vi "SetControlSpecific.vi"(7 "Dictionary":T2, 8 "error in (no error)":errorcluster, 9 "Font Info":T1, 10 "Target Language":string, 11 "Control Reference":refnum<vi>) -> (0 "error out":errorcluster, 3 "Control ref out":refnum<vi>)   [LabVIEW 2017, in "JKI Simple Localization.lvlib"]
uses:
  API/JKI Simple Localization.lvlib
  Definitions/Dictionary--Cluster.ctl
  Definitions/Private/FontCluster.ctl
  Definitions/Private/Phrase Dictionary.ctl
  Definitions/Private/Font Info.ctl
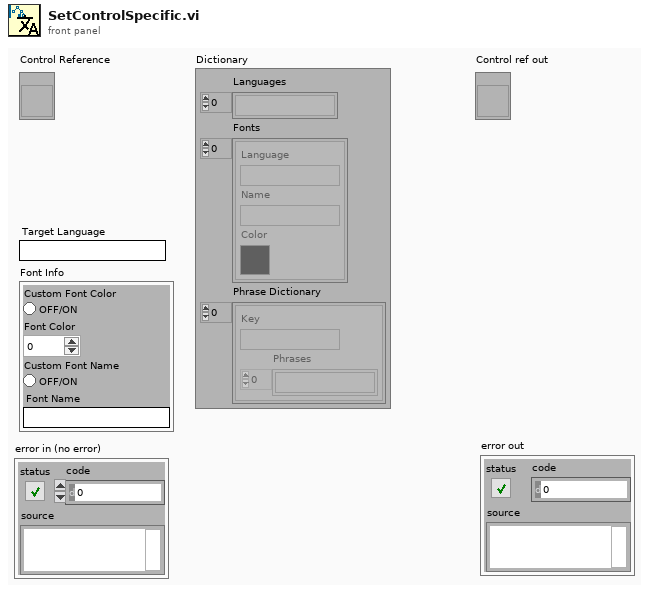
[diagram p1: front panel]
types:
  T1 = typedef "JKI Simple Localization.lvlib/Font Info.ctl" = cluster{"Custom Font Color":bool, "Font Color":u32, "Custom Font Name":bool, "Font Name":string}
  T2 = typedef "JKI Simple Localization.lvlib/Dictionary--Cluster.ctl" = cluster{"Languages":string[], "Fonts":T3[], "Phrase Dictionary":T4[]}
  T3 = typedef "JKI Simple Localization.lvlib/FontCluster.ctl" = cluster{"Language":string, "Name":string, "Color":u32}
  T4 = typedef "JKI Simple Localization.lvlib/Phrase Dictionary.ctl" = cluster{"Key":string, "Phrases":string[]}
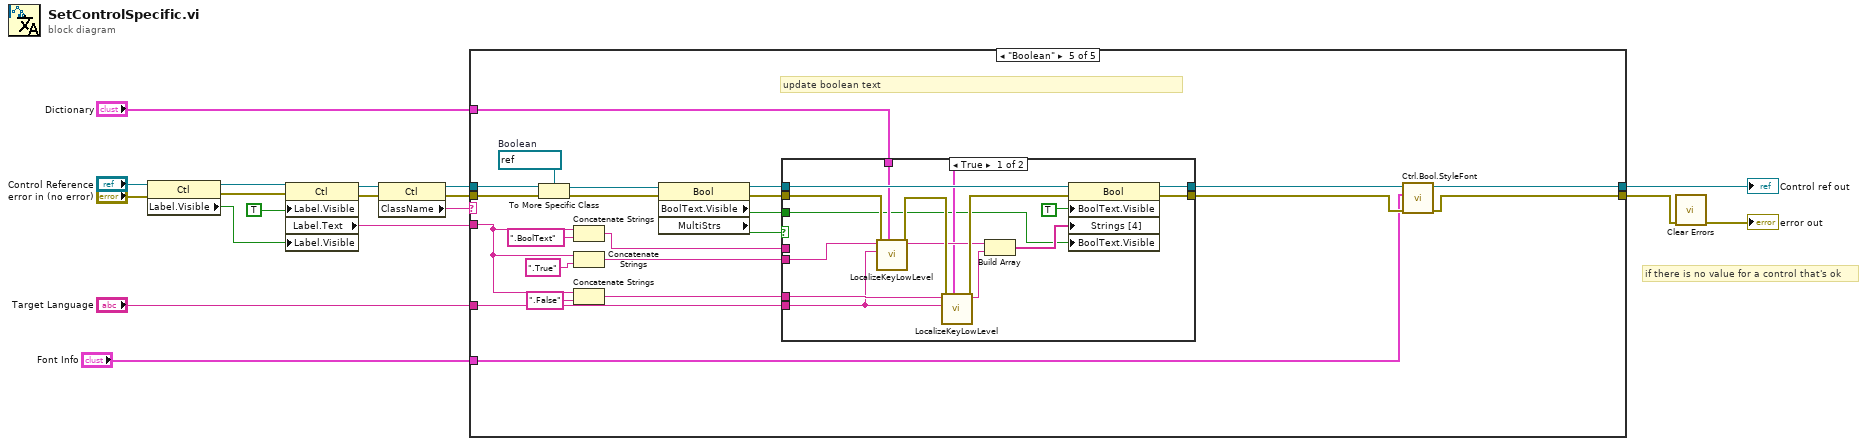
[diagram p0: block diagram]
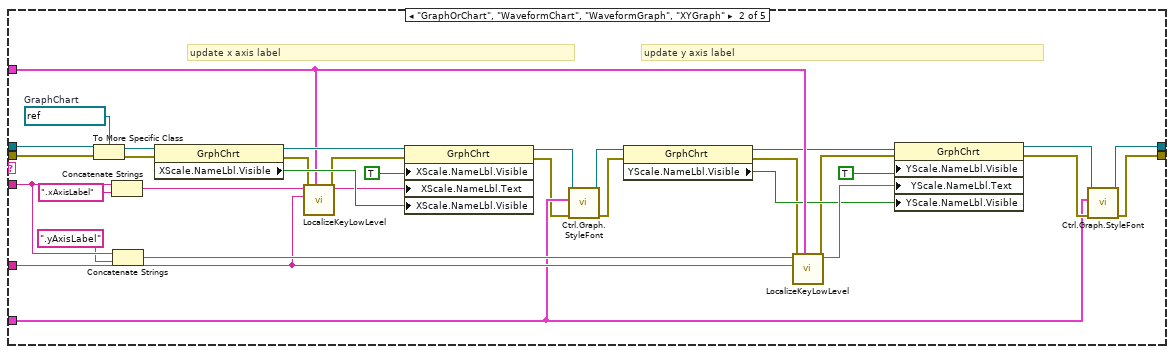
[diagram p3: hidden frame]
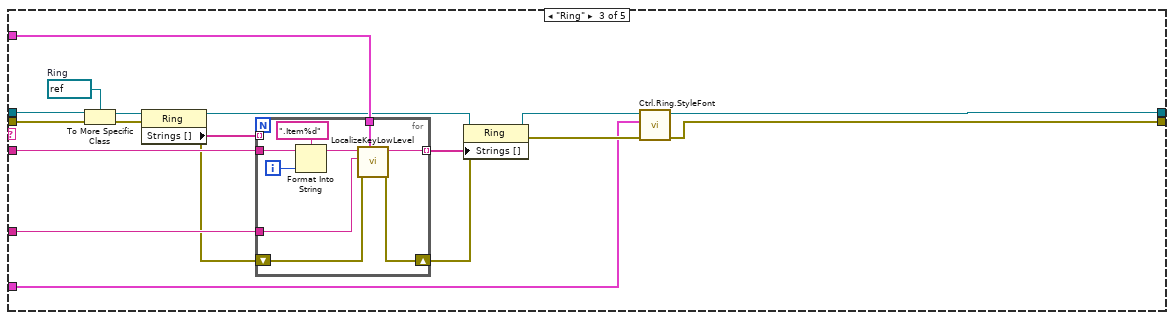
[diagram p4: hidden frame]
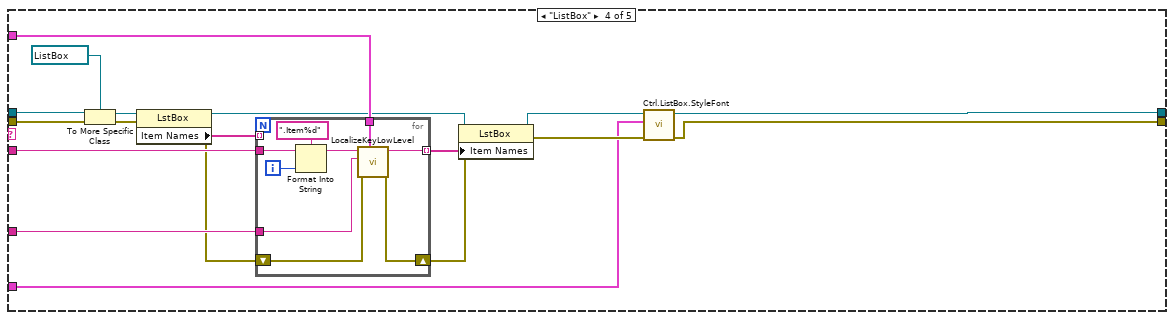
[diagram p5: hidden frame]
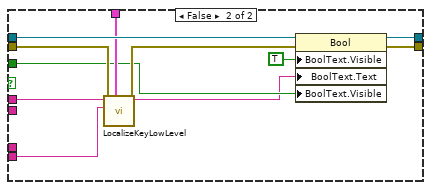
[diagram p6: hidden frame]
diagram:
  # "if there is no value for a control that's ok"
  n1 = property on="Property Node" class="Ctl"(reference="Control Reference", error in="error in (no error)") -> (reference out=w17:refnum<vi>, error out=w14:errorcluster, "Label.Visible"=w16:bool)
  n2 = property on="Property Node" class="Ctl"(reference=w17, error in=w14, "Label.Visible"=TRUE, "Label.Visible"=w16) -> (reference out=w12:refnum<vi>, error out=w8:errorcluster, "Label.Text"=w11:string)
  n3 = property on="Property Node" class="Ctl"(reference=w12, error in=w8) -> (reference out=w10:refnum<vi>, error out=w7:errorcluster, "ClassName"=w18:string)
  n4 = case shown="\"Boolean\"" w18 {
    tunnel: w11 -> [_ w44 w65 w93 w110]
    tunnel: w10 -> [w20 w52 w70 w98 w130]
    tunnel: "Dictionary" -> [_ w41 w64 w92 w121]
    tunnel: "Target Language" -> [_ w30 w63 w91 w118]
    tunnel: w7 -> [w19 w36 w69 w97 w124]
    tunnel: [w20 w26 w57 w83 w116] -> w6
    tunnel: [w19 w24 w55 w84 w114] -> w3
    tunnel: "Font Info" -> [_ w23 w54 w81 w113]
    frame "0", Default {
    }
    frame "GraphOrChart", "WaveformChart", "WaveformGraph", "XYGraph" {
      w50 = refnum<vi> refnum  # GraphChart
      # "update y axis label"
      # "update x axis label"
      n5 = To More Specific Class(target class=w50, reference=w52, error in=w36) -> (specific class reference=w51:refnum<vi>, error out=w35:errorcluster)
      n6 = Concatenate Strings(w44, ".xAxisLabel" ("string")) -> (w48:string)
      n7 = Concatenate Strings(w44, ".yAxisLabel" ("string")) -> (w42:string)
      n8 = property class="GrphChrt"(reference=w51, error in=w35) -> (reference out=w45:refnum<vi>, error out=w34:errorcluster, "XScale.NameLbl.Visible"=w49:bool)
      n9 = call "LocalizeKeyLowLevel.vi"("Dictionary"=w41, "error in (no error)"=w34, "Target Language"=w30, "Key"=w48) -> ("error out"=w33:errorcluster, "Localized Phrase"=w47:string)  [unwired: 6 in]
      n10 = property class="GrphChrt"(reference=w45, error in=w33, "XScale.NameLbl.Visible"=TRUE ("X Scale.Name Label.Visible"), "XScale.NameLbl.Text"=w47, "XScale.NameLbl.Visible"=w49) -> (reference out=w29:refnum<vi>, error out=w22:errorcluster)
      n11 = call "Ctrl.Graph.StyleFont.vi"("error in (no error)"=w22, "Font Info"=w23, "Graph Ctrl Ref in"=w29) -> ("error out"=w21:errorcluster, "Graph Ctrl Ref out"=w28:refnum<vi>)  [unwired: 7 in]
      n12 = property class="GrphChrt"(reference=w28, error in=w21) -> (reference out=w40:refnum<vi>, error out=w32:errorcluster, "YScale.NameLbl.Visible"=w37:bool)
      n13 = call "LocalizeKeyLowLevel.vi"("Dictionary"=w41, "error in (no error)"=w32, "Target Language"=w30, "Key"=w42) -> ("error out"=w31:errorcluster, "Localized Phrase"=w38:string)  [unwired: 6 in]
      n14 = property class="GrphChrt"(reference=w40, error in=w31, "YScale.NameLbl.Visible"=TRUE ("X Scale.Name Label.Visible"), "YScale.NameLbl.Text"=w38, "YScale.NameLbl.Visible"=w37) -> (reference out=w27:refnum<vi>, error out=w25:errorcluster)
      n15 = call "Ctrl.Graph.StyleFont.vi"("error in (no error)"=w25, "Font Info"=w23, "Graph Ctrl Ref in"=w27) -> ("error out"=w24:errorcluster, "Graph Ctrl Ref out"=w26:refnum<vi>)  [unwired: 7 in]
    }
    frame "Ring" {
      w71 = refnum<vi> refnum  # Ring
      n16 = To More Specific Class(target class=w71, reference=w70, error in=w69) -> (specific class reference=w68:refnum<vi>, error out=w67:errorcluster)
      n17 = property class="Ring"(reference=w68, error in=w67) -> (reference out=w61:refnum<vi>, error out=w60:errorcluster, "Strings []"=w66:string[])
      n18 = for {
        tunnel: w66 -> [_] mode=indexing
        tunnel: w65 -> [w80]
        tunnel: w64 -> [w77]
        shift-right: [w76] -> w59
        shift-left: w60 -> [w73]
        tunnel: w63 -> [w72]
        tunnel: [w74] -> w62 mode=indexing
        i -> [w78]
        n19 = Format Into String(format string=".Item%d", initial string=w80, w78) -> (resulting string=w75:string)  [unwired: 1 in, 1 out]
        n20 = call "LocalizeKeyLowLevel.vi"("Dictionary"=w77, "error in (no error)"=w73, "Target Language"=w72, "Key"=w75) -> ("error out"=w76:errorcluster, "Localized Phrase"=w74:string)  [unwired: 6 in]
      }
      n21 = property class="Ring"(reference=w61, error in=w59, "Strings []"=w62) -> (reference out=w58:refnum<vi>, error out=w56:errorcluster)
      n22 = call "Ctrl.Ring.StyleFont.vi"("error in (no error)"=w56, "Font Info"=w54, "Ring Ref in"=w58) -> ("error out"=w55:errorcluster, "Ring Ref out"=w57:refnum<vi>)  [unwired: 7 in]
    }
    frame "ListBox" {
      n23 = To More Specific Class(target class=refnum<vi> refnum ("reference out"), reference=w98, error in=w97) -> (specific class reference=w96:refnum<vi>, error out=w95:errorcluster)
      n24 = property class="LstBox"(reference=w96, error in=w95) -> (reference out=w89:refnum<vi>, error out=w88:errorcluster, "Item Names"=w94:string[])
      n25 = for {
        tunnel: w94 -> [_] mode=indexing
        tunnel: w93 -> [w107]
        tunnel: w92 -> [w104]
        shift-right: [w103] -> w87
        shift-left: w88 -> [w100]
        tunnel: w91 -> [w99]
        tunnel: [w101] -> w90 mode=indexing
        i -> [w105]
        n26 = Format Into String(format string=".Item%d", initial string=w107, w105) -> (resulting string=w102:string)  [unwired: 1 in, 1 out]
        n27 = call "LocalizeKeyLowLevel.vi"("Dictionary"=w104, "error in (no error)"=w100, "Target Language"=w99, "Key"=w102) -> ("error out"=w103:errorcluster, "Localized Phrase"=w101:string)  [unwired: 6 in]
      }
      n28 = property class="LstBox"(reference=w89, error in=w87, "Item Names"=w90) -> (reference out=w82:refnum<vi>, error out=w85:errorcluster)
      n29 = call "Ctrl.ListBox.StyleFont.vi"("error in (no error)"=w85, "Font Info"=w81, "Listbox Ref"=w82) -> ("error out"=w84:errorcluster, "Listbox Ref out"=w83:refnum<vi>)  [unwired: 7 in]
    }
    frame "Boolean" {
      w128 = refnum<vi> refnum  # Boolean
      # "update boolean text"
      n30 = To More Specific Class(target class=w128, reference=w130, error in=w124) -> (specific class reference=w129:refnum<vi>, error out=w123:errorcluster)
      n31 = Concatenate Strings(w110, ".BoolText" ("string")) -> (w108:string)
      n32 = Concatenate Strings(w110, ".True" ("string")) -> (w127:string)
      n33 = Concatenate Strings(w110, ".False" ("string")) -> (w125:string)
      n34 = property class="Bool"(reference=w129, error in=w123) -> (reference out=w126:refnum<vi>, error out=w122:errorcluster, "BoolText.Visible"=w120:bool, "MultiStrs"=w119:bool)
      n35 = case shown="True" w119 {
        tunnel: w127 -> [w145 _]
        tunnel: w126 -> [w144 w156]
        tunnel: w125 -> [w143 _]
        tunnel: w118 -> [w131 w146]
        tunnel: w122 -> [w142 w155]
        tunnel: w121 -> [w137 w153]
        tunnel: w120 -> [w134 w151]
        tunnel: w108 -> [_ w150]
        tunnel: [w133 w148] -> w117
        tunnel: [w132 w147] -> w115
        frame True {
          n36 = call "LocalizeKeyLowLevel.vi"("Dictionary"=w137, "error in (no error)"=w142, "Target Language"=w131, "Key"=w145) -> ("error out"=w141:errorcluster, "Localized Phrase"=w139:string)  [unwired: 6 in]
          n37 = call "LocalizeKeyLowLevel.vi"("Dictionary"=w137, "error in (no error)"=w141, "Target Language"=w131, "Key"=w143) -> ("error out"=w140:errorcluster, "Localized Phrase"=w138:string)  [unwired: 6 in]
          n38 = Build Array(w139, w138) -> (w136:string[])
          n39 = property class="Bool"(reference=w144, error in=w140, "BoolText.Visible"=TRUE ("X Scale.Name Label.Visible"), "Strings [4]"=w136, "BoolText.Visible"=w134) -> (reference out=w133:refnum<vi>, error out=w132:errorcluster)
        }
        frame False {
          n40 = call "LocalizeKeyLowLevel.vi"("Dictionary"=w153, "error in (no error)"=w155, "Target Language"=w146, "Key"=w150) -> ("error out"=w154:errorcluster, "Localized Phrase"=w149:string)  [unwired: 6 in]
          n41 = property class="Bool"(reference=w156, error in=w154, "BoolText.Visible"=TRUE ("X Scale.Name Label.Visible"), "BoolText.Text"=w149, "BoolText.Visible"=w151) -> (reference out=w148:refnum<vi>, error out=w147:errorcluster)
        }
      }
      n42 = call "Ctrl.Bool.StyleFont.vi"("error in (no error)"=w115, "Font Info"=w113, "Bool Ref in"=w117) -> ("error out"=w114:errorcluster, "Bool Ref out"=w116:refnum<vi>)  [unwired: 7 in]
    }
  }
  "Control ref out" <- w6
  n43 = call <vilib>:"Clear Errors.vi"("error in (no error)"=w3) -> ("error out"=→"error out":errorcluster)  [unwired: 5 in, 1 out]
